vi "Timing Pour's.vi"(8 "Error In Global Timing":errorcluster, 11 "Timing Command":enum16{"Reset", "Stop", "Start"}(ring)) -> (0 "Error Out Global Timing":errorcluster, 1 "TimeStamp Read":timestamp, 3 "Seconds Passed":dbl)   [LabVIEW 2020]
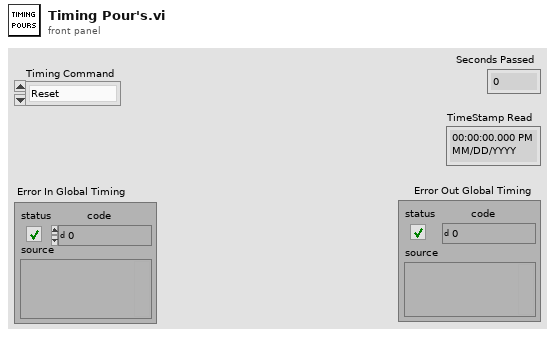
[diagram p1: front panel]
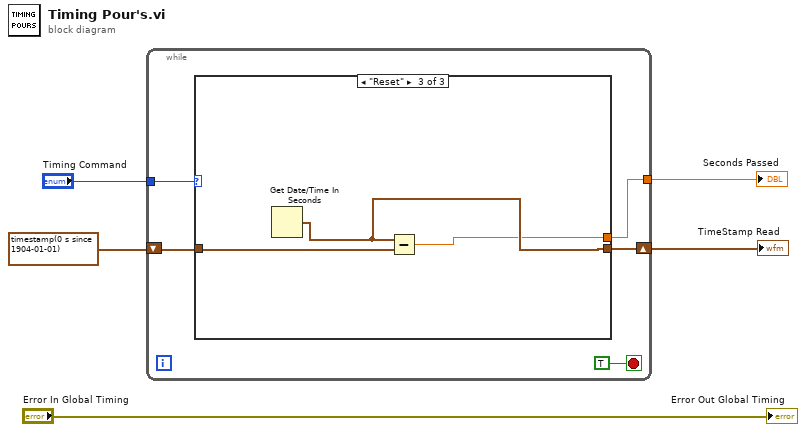
[diagram p0: block diagram]
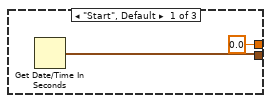
[diagram p2: hidden frame]
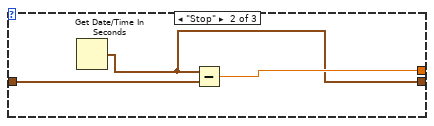
[diagram p3: hidden frame]
diagram:
  n1 = while {
    tunnel: "Timing Command" -> [w10]
    shift-right: [w7] -> w2
    shift-left: timestamp(0 s since 1904-01-01) -> [w8]
    tunnel: [w6] -> w3
    stop <- TRUE stop-if-true
    n2 = case shown="\"Reset\"" w10 {
      tunnel: w8 -> [_ w15 w16]
      tunnel: [w12 w13 w18] -> w7
      tunnel: [0.0 w14 w17] -> w6
      frame "Start", Default {
        n3 = Get Date/Time In Seconds() -> (seconds since 1Jan1904=w12:timestamp)
      }
      frame "Stop" {
        n4 = Get Date/Time In Seconds() -> (seconds since 1Jan1904=w13:timestamp)
        n5 = Subtract(x=w13, y=w15) -> (x-y=w14:dbl)
      }
      frame "Reset" {
        n6 = Get Date/Time In Seconds() -> (seconds since 1Jan1904=w18:timestamp)
        n7 = Subtract(x=w18, y=w16) -> (x-y=w17:dbl)
      }
    }
  }
  "Seconds Passed" <- w3
  "TimeStamp Read" <- w2
  "Error Out Global Timing" <- "Error In Global Timing"
